vi "fake_rotate_instability.vi"(0 "rotation":cluster{"pitch":dbl, "roll":dbl, "yaw":dbl}={"pitch"=18.0, "roll"=0.0, "yaw"=-4.0}, 1 "stabile":bool) -> (2 "Pitch":dbl=18.0, 3 "Roll":dbl, 4 "Yow":dbl=-4.0)   [LabVIEW 2017]
uses:
  <vilib>/Analysis/baseanly.llb/Real Dot Product.vi
  <vilib>/Analysis/NI_AALBase.lvlib
panel:
  in  "old rotation":cluster{"pitch":dbl, "roll":dbl, "yaw":dbl}[](array[cluster])=[{"pitch"=29.0, "roll"=4.0, "yaw"=11.0}, {"pitch"=29.0, "roll"=4.0, "yaw"=11.0}, {"pitch"=29.0, "roll"=4.0, "yaw"=11.0}, {"pitch"=29.0, "roll"=4.0, "yaw"=11.0}, {"pitch"=29.0, "roll"=4.0, "yaw"=11.0}, {"pitch"=29.0, "roll"=4.0, "yaw"=11.0}, {"pitch"=29.0, "roll"=4.0, "yaw"=11.0}, {"pitch"=29.0, "roll"=4.0, "yaw"=11.0}, {"pitch"=29.0, "roll"=4.0, "yaw"=11.0}]
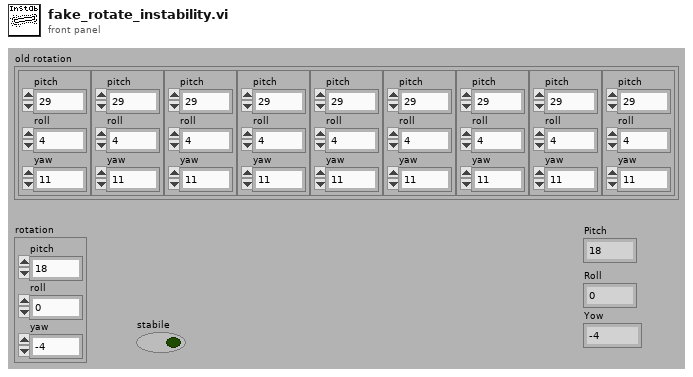
[diagram p1: front panel]
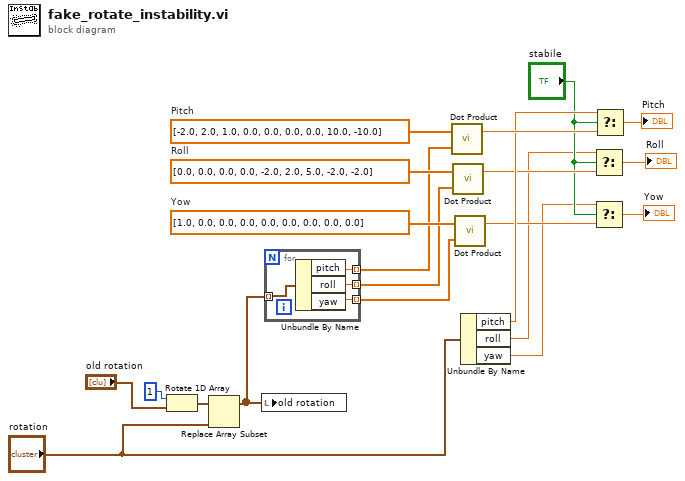
[diagram p0: block diagram]
diagram:
  w19 = dbl[] [1.0, 0.0, 0.0, 0.0, 0.0, 0.0, 0.0, 0.0, 0.0]  # Yow
  w17 = dbl[] [0.0, 0.0, 0.0, 0.0, -2.0, 2.0, 5.0, -2.0, -2.0]  # Roll
  w16 = dbl[] [-2.0, 2.0, 1.0, 0.0, 0.0, 0.0, 0.0, 10.0, -10.0]  # Pitch
  n1 = Rotate 1D Array(1:"old rotation", 2:1 ("n")) -> (0:w13:cluster{"pitch":dbl, "roll":dbl, "yaw":dbl}[])
  n2 = Replace Array Subset(array=w13, new element="rotation") -> (w11:cluster{"pitch":dbl, "roll":dbl, "yaw":dbl}[])  [unwired: 1 in]
  n3 = local write "old rotation"(w11) -> ()
  n4 = for {
    tunnel: w11 -> [w25] mode=indexing
    tunnel: [w24] -> w15 mode=indexing
    tunnel: [w23] -> w18 mode=indexing
    tunnel: [w22] -> w20 mode=indexing
    n5 = Unbundle By Name(w25) -> ("pitch"=w24:dbl, "roll"=w23:dbl, "yaw"=w22:dbl)
  }
  n6 = call-poly <vilib>:"Dot Product.vi"("Y Vector"=w15, "X Vector"=w16) -> ("X * Y"=w21:dbl)  [unwired: 1 out]
  n7 = call-poly <vilib>:"Dot Product.vi"("Y Vector"=w18, "X Vector"=w17) -> ("X * Y"=w4:dbl)  [unwired: 1 out]
  n8 = call-poly <vilib>:"Dot Product.vi"("Y Vector"=w20, "X Vector"=w19) -> ("X * Y"=w5:dbl)  [unwired: 1 out]
  n9 = Unbundle By Name("rotation") -> ("pitch"=w6:dbl, "roll"=w2:dbl, "yaw"=w1:dbl)
  n10 = Select(t=w2, s="stabile", f=w4) -> (s? t:f=→"Roll":dbl)
  n11 = Select(t=w1, s="stabile", f=w5) -> (s? t:f=→"Yow":dbl)
  n12 = Select(t=w6, s="stabile", f=w21) -> (s? t:f=→"Pitch":dbl)
